vi "selectTrigger.vi"(3 "triggerEdge":T1=enum."true-false", 4 "MCSSelectTrigger":T2) -> (1 "fired":bool)   [LabVIEW 2014]
uses:
  Controls/selectTrigger.ctl
  Controls/triggerEdge.ctl
  <vilib>/rvi/eio/common/nirviEmuTemplateMethod_errors.vi
  <vilib>/eio/EIONode/EIONode.xnode
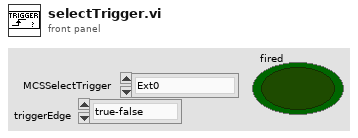
[diagram p1: front panel]
types:
  T1 = typedef "triggerEdge.ctl" = enum8{"either", "false-true", "true-false"}
  T2 = typedef "selectTrigger.ctl" = enum8{"Ext0", "Ext1", "Ext2", "Ext3", "Ext4", "Ext5", "Ext6", "Ext7", "Int0", "Int1", "Int2", "Int3", "Int4", "Int5", "Int6", "Int7"}
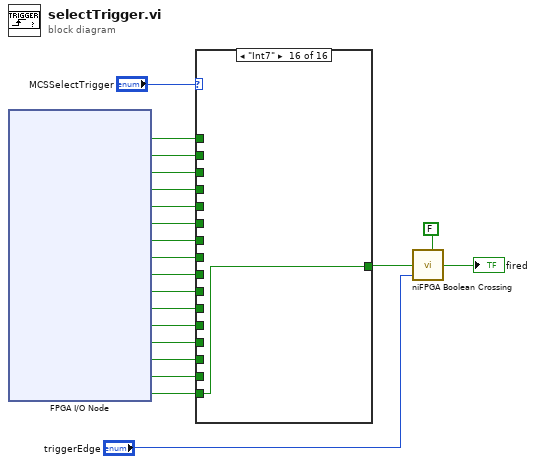
[diagram p0: block diagram]
diagram:
  n1 = xnode "FPGA I/O Node"() -> ("Connector1/DIO24"=w20:bool, "Connector1/DIO25"=w19:bool, "Connector1/DIO26"=w18:bool, "Connector1/DIO27"=w17:bool, "Connector1/DIO28"=w16:bool, "Connector1/DIO29"=w15:bool, "Connector1/DIO30"=w14:bool, "Connector1/DIO31"=w13:bool, "PXI_Trig0"=w12:bool, "PXI_Trig1"=w11:bool, "PXI_Trig2"=w10:bool, "PXI_Trig3"=w9:bool, "PXI_Trig4"=w8:bool, "PXI_Trig5"=w7:bool, "PXI_Trig6"=w6:bool, "PXI_Trig7"=w5:bool)  [unwired: 16 in, 16 out]
  n2 = case shown="\"Int7\"" "MCSSelectTrigger" {
    tunnel: w20 -> [w22 _ _ _ _ _ _ _ _ _ _ _ _ _ _ _]
    tunnel: w19 -> [_ w23 _ _ _ _ _ _ _ _ _ _ _ _ _ _]
    tunnel: w18 -> [_ _ w24 _ _ _ _ _ _ _ _ _ _ _ _ _]
    tunnel: w17 -> [_ _ _ w25 _ _ _ _ _ _ _ _ _ _ _ _]
    tunnel: w16 -> [_ _ _ _ w26 _ _ _ _ _ _ _ _ _ _ _]
    tunnel: w15 -> [_ _ _ _ _ w27 _ _ _ _ _ _ _ _ _ _]
    tunnel: w14 -> [_ _ _ _ _ _ w28 _ _ _ _ _ _ _ _ _]
    tunnel: w13 -> [_ _ _ _ _ _ _ w29 _ _ _ _ _ _ _ _]
    tunnel: w12 -> [_ _ _ _ _ _ _ _ w30 _ _ _ _ _ _ _]
    tunnel: w11 -> [_ _ _ _ _ _ _ _ _ w31 _ _ _ _ _ _]
    tunnel: w10 -> [_ _ _ _ _ _ _ _ _ _ w32 _ _ _ _ _]
    tunnel: w9 -> [_ _ _ _ _ _ _ _ _ _ _ w33 _ _ _ _]
    tunnel: w8 -> [_ _ _ _ _ _ _ _ _ _ _ _ w34 _ _ _]
    tunnel: w7 -> [_ _ _ _ _ _ _ _ _ _ _ _ _ w35 _ _]
    tunnel: w6 -> [_ _ _ _ _ _ _ _ _ _ _ _ _ _ w36 _]
    tunnel: w5 -> [_ _ _ _ _ _ _ _ _ _ _ _ _ _ _ w37]
    tunnel: [w22 w23 w24 w25 w26 w27 w28 w29 w30 w31 w32 w33 w34 w35 w36 w37] -> w4
    frame "Ext0", Default {
    }
    frame "Ext1" {
    }
    frame "Ext2" {
    }
    frame "Ext3" {
    }
    frame "Ext4" {
    }
    frame "Ext5" {
    }
    frame "Ext6" {
    }
    frame "Ext7" {
    }
    frame "Int0" {
    }
    frame "Int1" {
    }
    frame "Int2" {
    }
    frame "Int3" {
    }
    frame "Int4" {
    }
    frame "Int5" {
    }
    frame "Int6" {
    }
    frame "Int7" {
    }
  }
  n3 = call <vilib>:"niFPGA Boolean Crossing.vi"("input"=w4, "triggerEdge"="triggerEdge", "initialize"=FALSE) -> ("crossing"=→"fired":bool)  [unwired: 6 in]
